vi "Build Map from Page GUIDs to Page VIs.vi"() -> (3 "page map GUID to VI ref":map{string, refnum<vi>}(c390))   [LabVIEW 2020, in "AIM MIL-STD-1553 System Explorer.lvlib" / "Implementation.lvlib" / "System Explorer Dispatcher.lvclass"]
uses:
  System Explorer Dispatcher.lvclass
  Scripting/Constants.vi
  System Explorer/Pages/Logging.vi
  Implementation.lvlib
  Scripting/AIM MIL-STD-1553 Scripting.lvlib
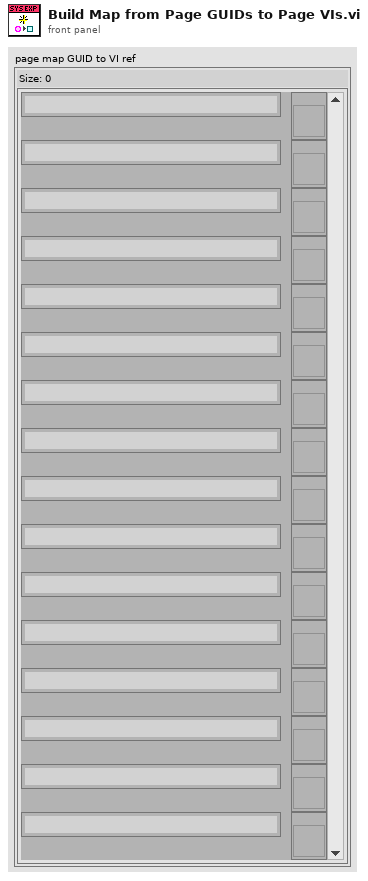
[diagram p1: front panel]
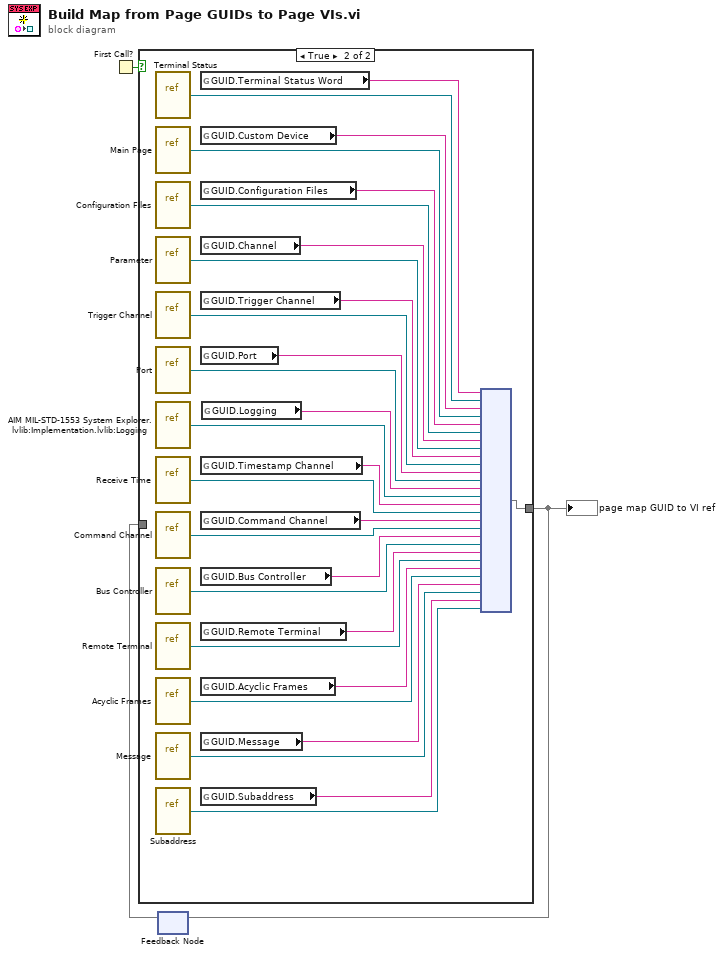
[diagram p0: block diagram]
diagram:
  n1 = First Call?() -> (First Call?: T/F=w1:bool)
  n2 = feedback #1() -> (w2:map{string, refnum<vi>})  [unwired: 1 in]
  n3 = case shown="True" w1 {
    tunnel: [w4 w33] -> w3
    tunnel: w2 -> [w4 _]
    frame False {
    }
    frame True {
      n4 = vi-ref "Terminal Status.vi"() -> (w6:refnum<vi>)
      n5 = vi-ref "Main Page.vi"() -> (w32:refnum<vi>)
      n6 = vi-ref "Configuration Files.vi"() -> (w30:refnum<vi>)
      n7 = vi-ref "Parameter.vi"() -> (w27:refnum<vi>)
      n8 = vi-ref "Trigger Channel.vi"() -> (w25:refnum<vi>)
      n9 = vi-ref "Port.vi"() -> (w23:refnum<vi>)
      n10 = vi-ref "AIM MIL-STD-1553 System Explorer.lvlib:Implementation.lvlib:Logging.vi"() -> (w21:refnum<vi>)
      n11 = vi-ref "Receive Time.vi"() -> (w19:refnum<vi>)
      n12 = vi-ref "Command Channel.vi"() -> (w17:refnum<vi>)
      n13 = vi-ref "Bus Controller.vi"() -> (w15:refnum<vi>)
      n14 = vi-ref "Remote Terminal.vi"() -> (w13:refnum<vi>)
      n15 = vi-ref "Acyclic Frames.vi"() -> (w11:refnum<vi>)
      n16 = vi-ref "Message.vi"() -> (w9:refnum<vi>)
      n17 = vi-ref "Subaddress.vi"() -> (w7:refnum<vi>)
      n18 = global read "Constants.vi" "GUID.Terminal Status Word"() -> (w5:string)
      n19 = global read "Constants.vi" "GUID.Custom Device"() -> (w31:string)
      n20 = global read "Constants.vi" "GUID.Configuration Files"() -> (w29:string)
      n21 = global read "Constants.vi" "GUID.Channel"() -> (w28:string)
      n22 = global read "Constants.vi" "GUID.Trigger Channel"() -> (w26:string)
      n23 = global read "Constants.vi" "GUID.Port"() -> (w24:string)
      n24 = global read "Constants.vi" "GUID.Timestamp Channel"() -> (w20:string)
      n25 = global read "Constants.vi" "GUID.Command Channel"() -> (w18:string)
      n26 = global read "Constants.vi" "GUID.Bus Controller"() -> (w16:string)
      n27 = global read "Constants.vi" "GUID.Remote Terminal"() -> (w14:string)
      n28 = global read "Constants.vi" "GUID.Acyclic Frames"() -> (w12:string)
      n29 = global read "Constants.vi" "GUID.Message"() -> (w10:string)
      n30 = global read "Constants.vi" "GUID.Subaddress"() -> (w8:string)
      n31 = global read "Constants.vi" "GUID.Logging"() -> (w22:string)
      n32 = node(w5, w6, w31, w32, w29, w30, w28, w27, w26, w25, w24, w23, w22, w21, w20, w19, w18, w17, w16, w15, w14, w13, w12, w11, w10, w9, w8, w7) -> (w33:map{string, refnum<vi>})
    }
  }
  "page map GUID to VI ref" <- w3
  n33 = feedback-in #1(w3) -> ()
